vi "rmad aux data to file.vi"(1 "Avalanch JBV":T1(array[cluster]) {"A2 mean" format="%.1f"; "A1 mean" format="%.1f"; "A1 std" format="%.1f"; "A2 std" format="%.1f"}, 2 "aux_datadir":string, 3 "event_datadir":string, 5 "Avalanch Packets":T3(array[cluster]) {"A1 std" format="%.1g"; "A2 std" format="%.1g"; "A3 std" format="%.1g"; "A4 std" format="%.1g"}, 7 "vdv_datadir":string, 9 "last packet type":u8[](array[numeric]), 11 "error in":errorcluster, 12 "AUX data":T2(array[cluster]) {"batteri (V)" format="%.3g"; "temperatur (c)" format="%.1g"}, 13 "mac adresses":T4) -> (15 "error out":errorcluster)   [LabVIEW 2017]
panel:
  out "previous line in dat file":string
  out "last vdv record number":i32
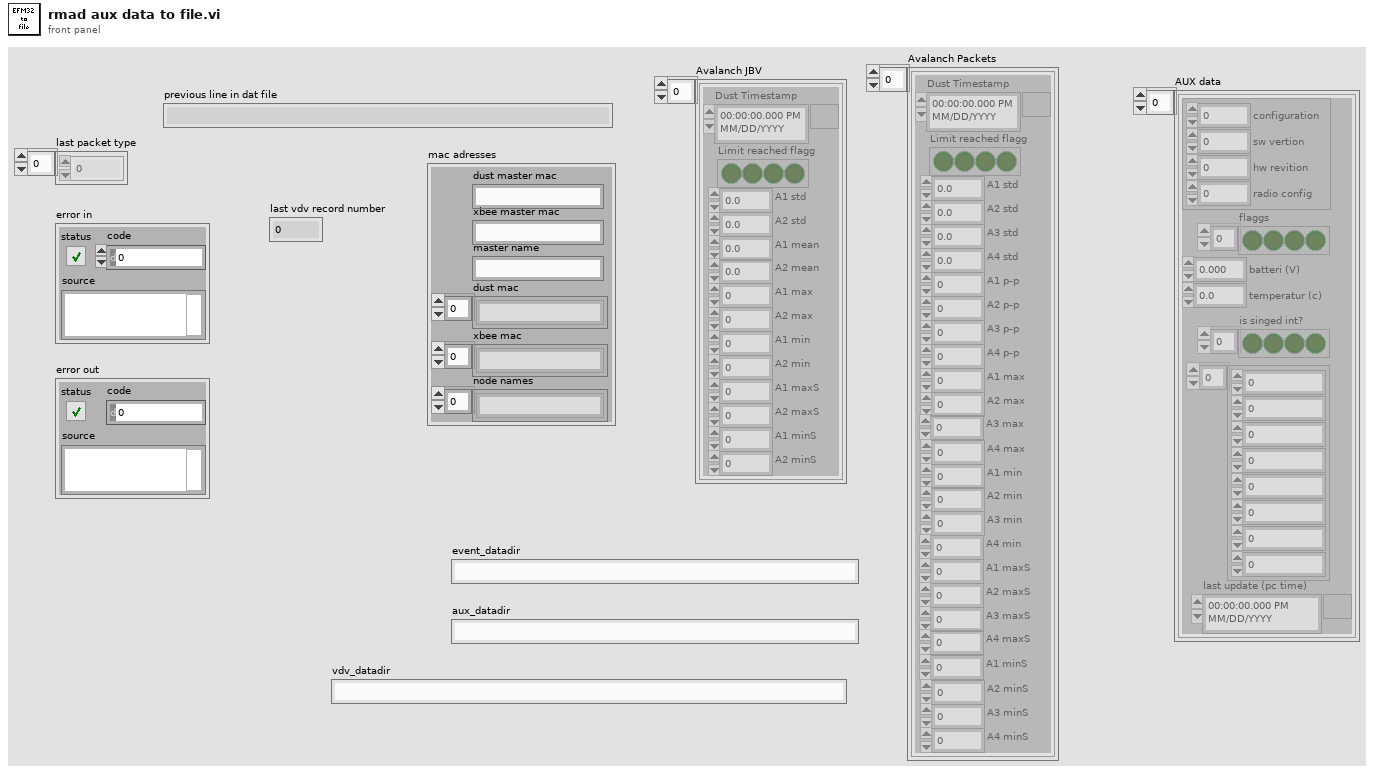
[diagram p1: front panel]
types:
  T1 = cluster{"Dust Timestamp":timestamp, "Limit reached flagg":bool[], "A1 std":sgl, "A2 std":sgl, "A1 mean":sgl, "A2 mean":sgl, "A1 max":i32, "A2 max":i32, "A1 min":i32, "A2 min":i32, "A1 maxS":u16, "A2 maxS":u16, "A1 minS":u16, "A2 minS":u16}[]
  T2 = cluster{cluster{"configuration":u8, "sw vertion":u8, "hw revition":u8, "radio config":u8}, "flaggs":bool[], "batteri (V)":dbl, "temperatur (c)":dbl, "is singed int?":bool[], dbl[], "last update (pc time)":timestamp}[]
  T3 = cluster{"Dust Timestamp":timestamp, "Limit reached flagg":bool[], "A1 std":sgl, "A2 std":sgl, "A3 std":sgl, "A4 std":sgl, "A1 p-p":sgl, "A2 p-p":sgl, "A3 p-p":sgl, "A4 p-p":sgl, "A1 max":u16, "A2 max":u16, "A3 max":u16, "A4 max":u16, "A1 min":u16, "A2 min":u16, "A3 min":u16, "A4 min":u16, "A1 maxS":u16, "A2 maxS":u16, "A3 maxS":u16, "A4 maxS":u16, "A1 minS":u16, "A2 minS":u16, "A3 minS":u16, "A4 minS":u16}[]
  T4 = cluster{"dust master mac":string, "xbee master mac":string, "master name":string, "dust mac":string[], "xbee mac":string[], "node names":string[]}
  T5 = enum16{"open", "replace", "create", "open or create", "replace or create", "replace or create with confirmation"}
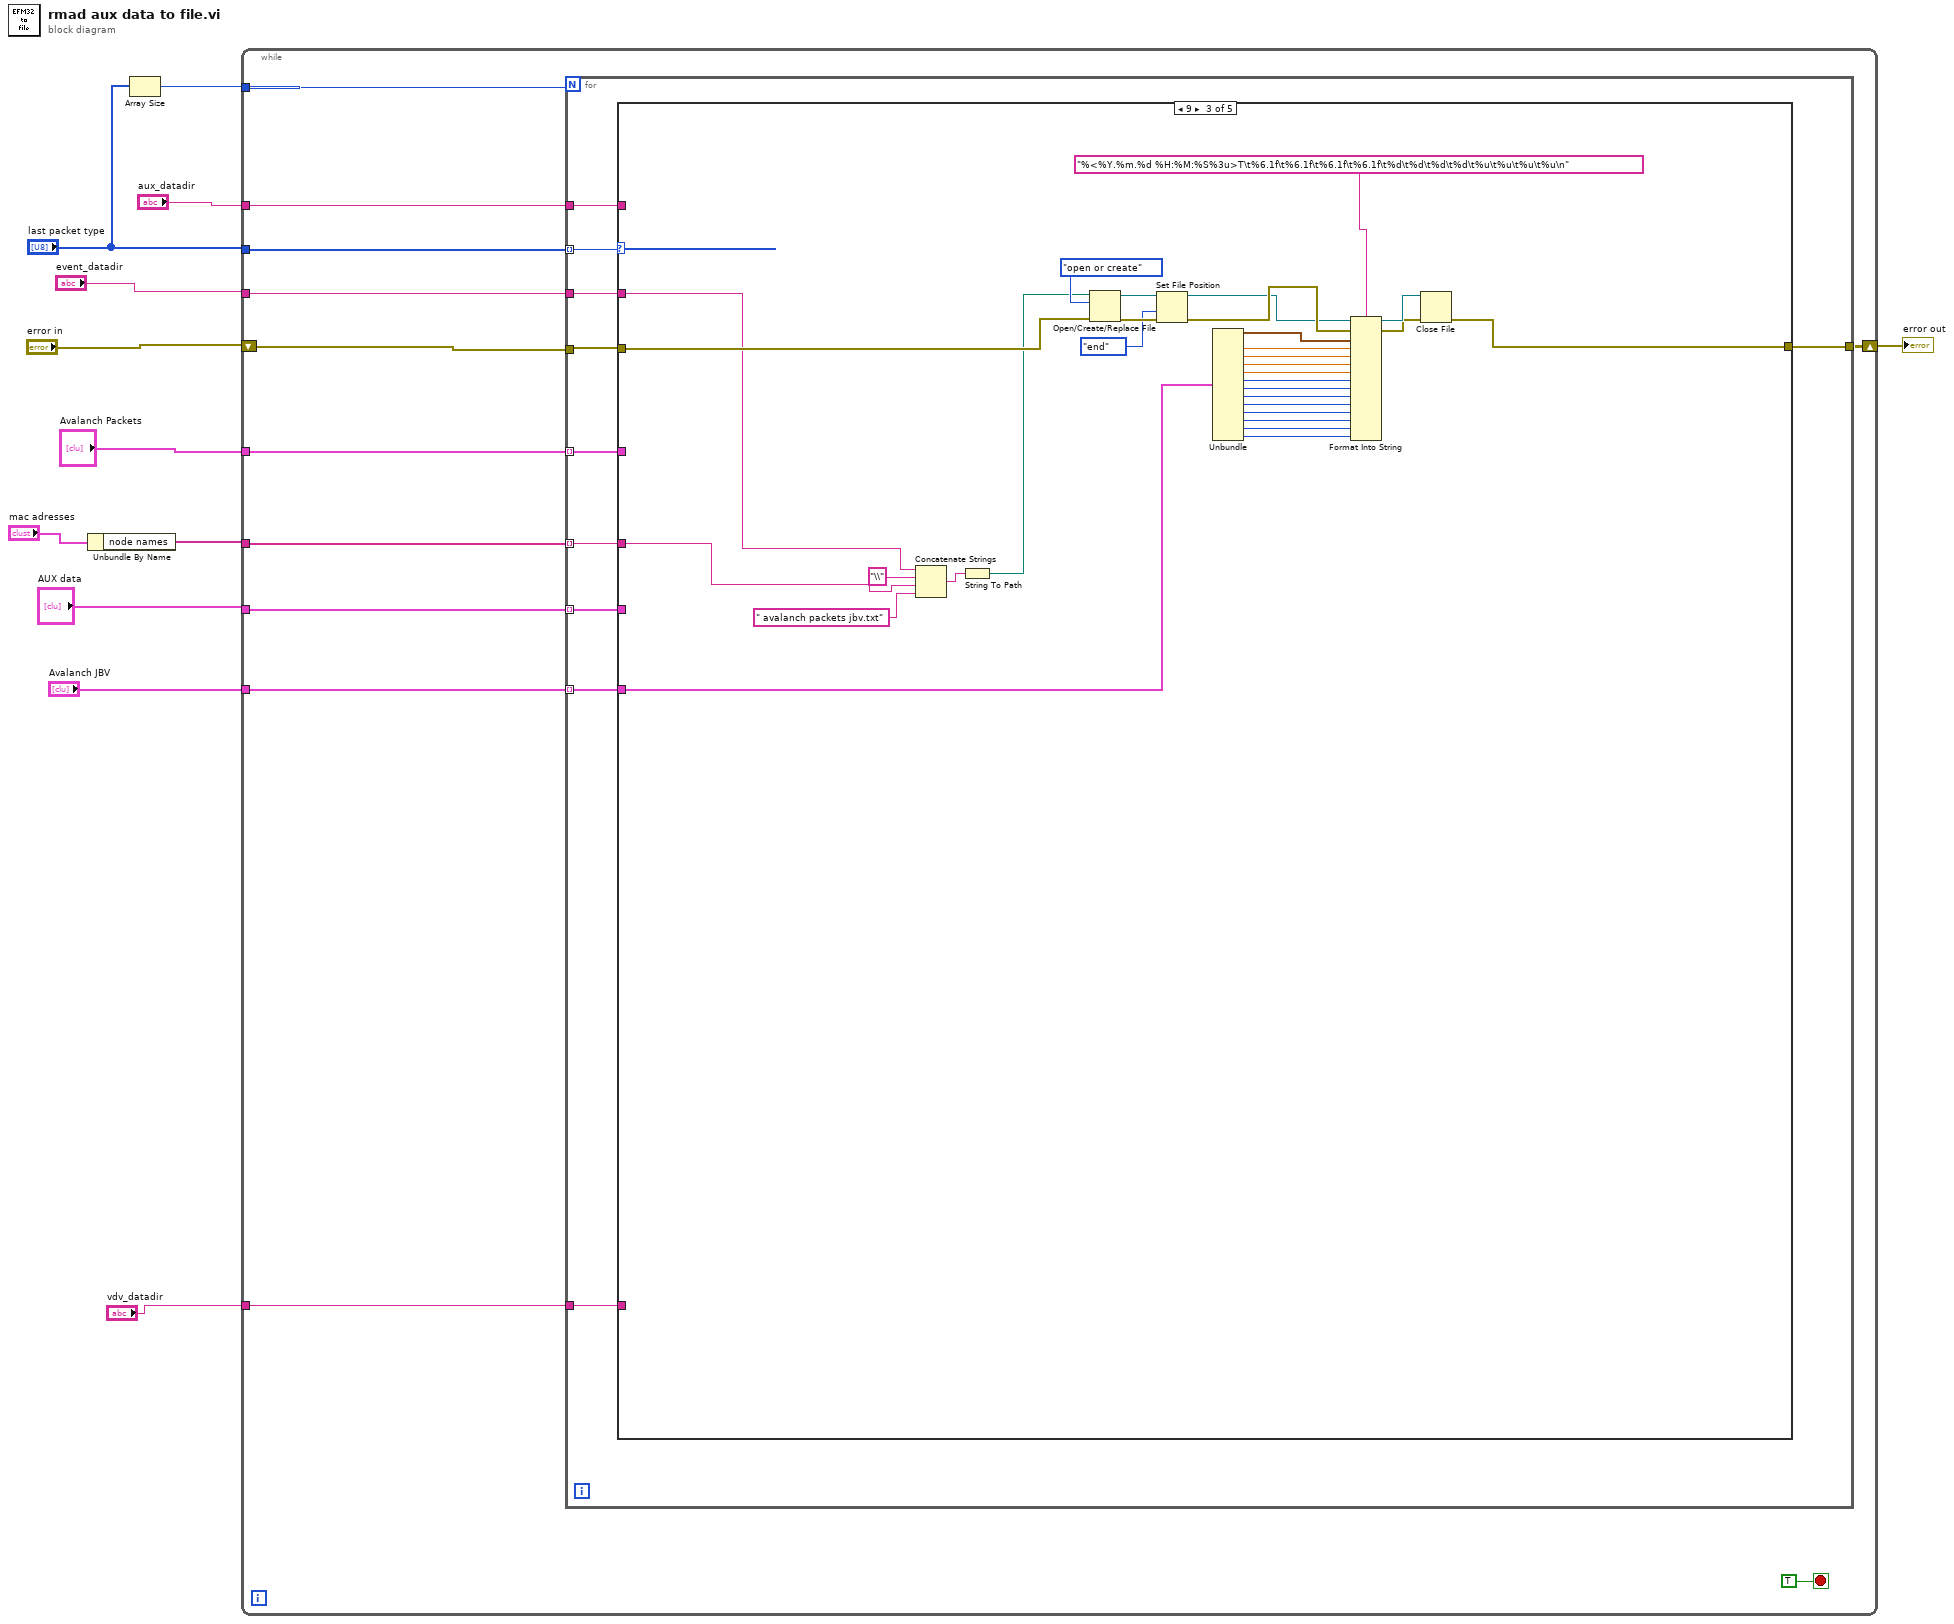
[diagram p0: block diagram]
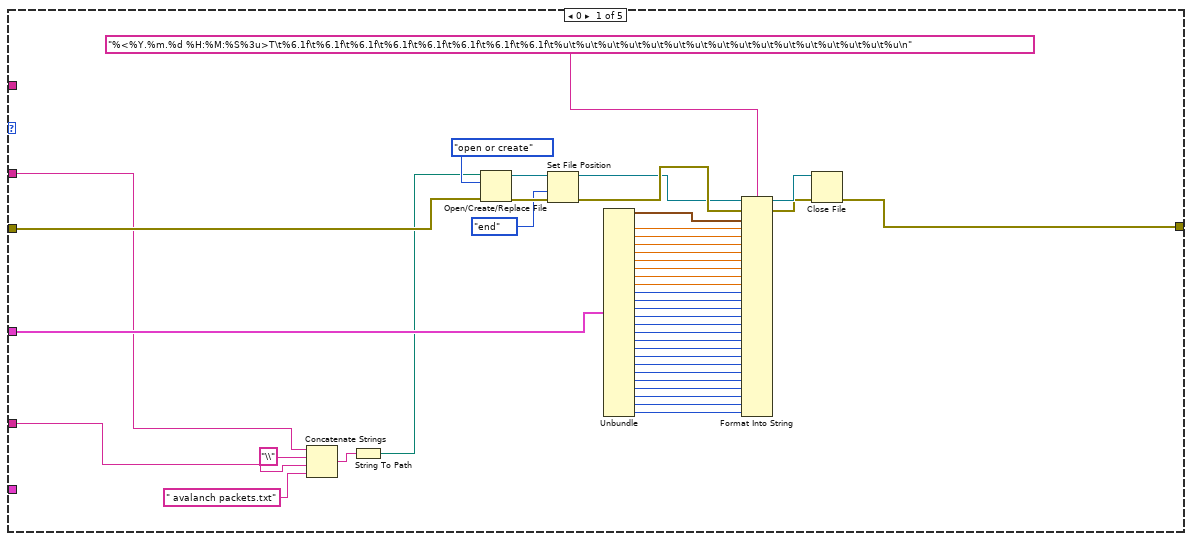
[diagram p2: hidden frame]
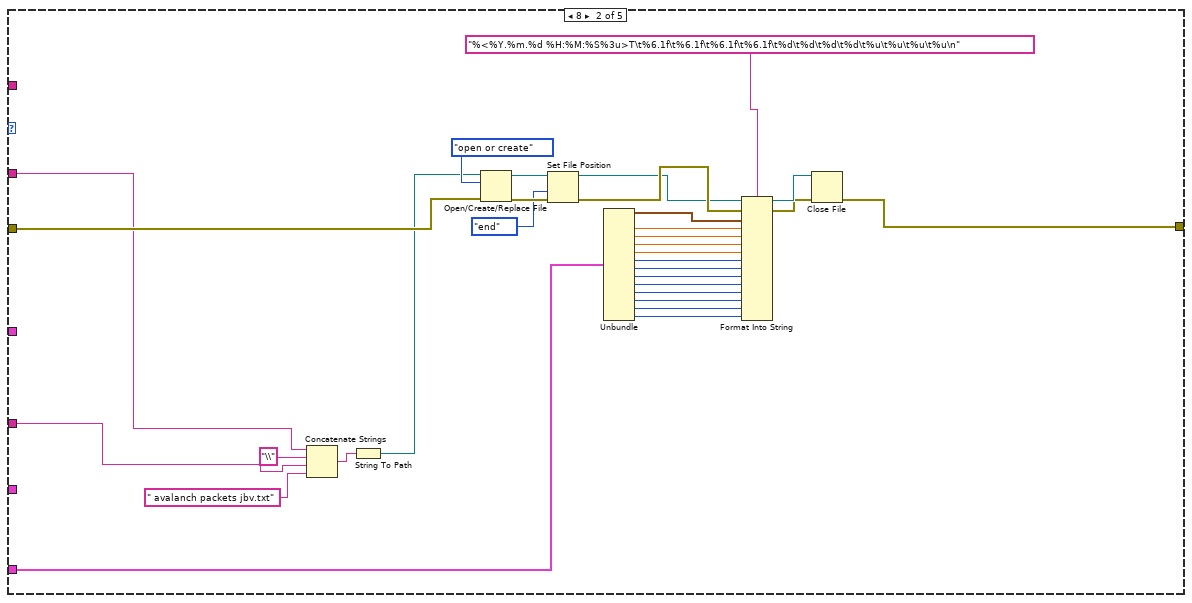
[diagram p3: hidden frame]
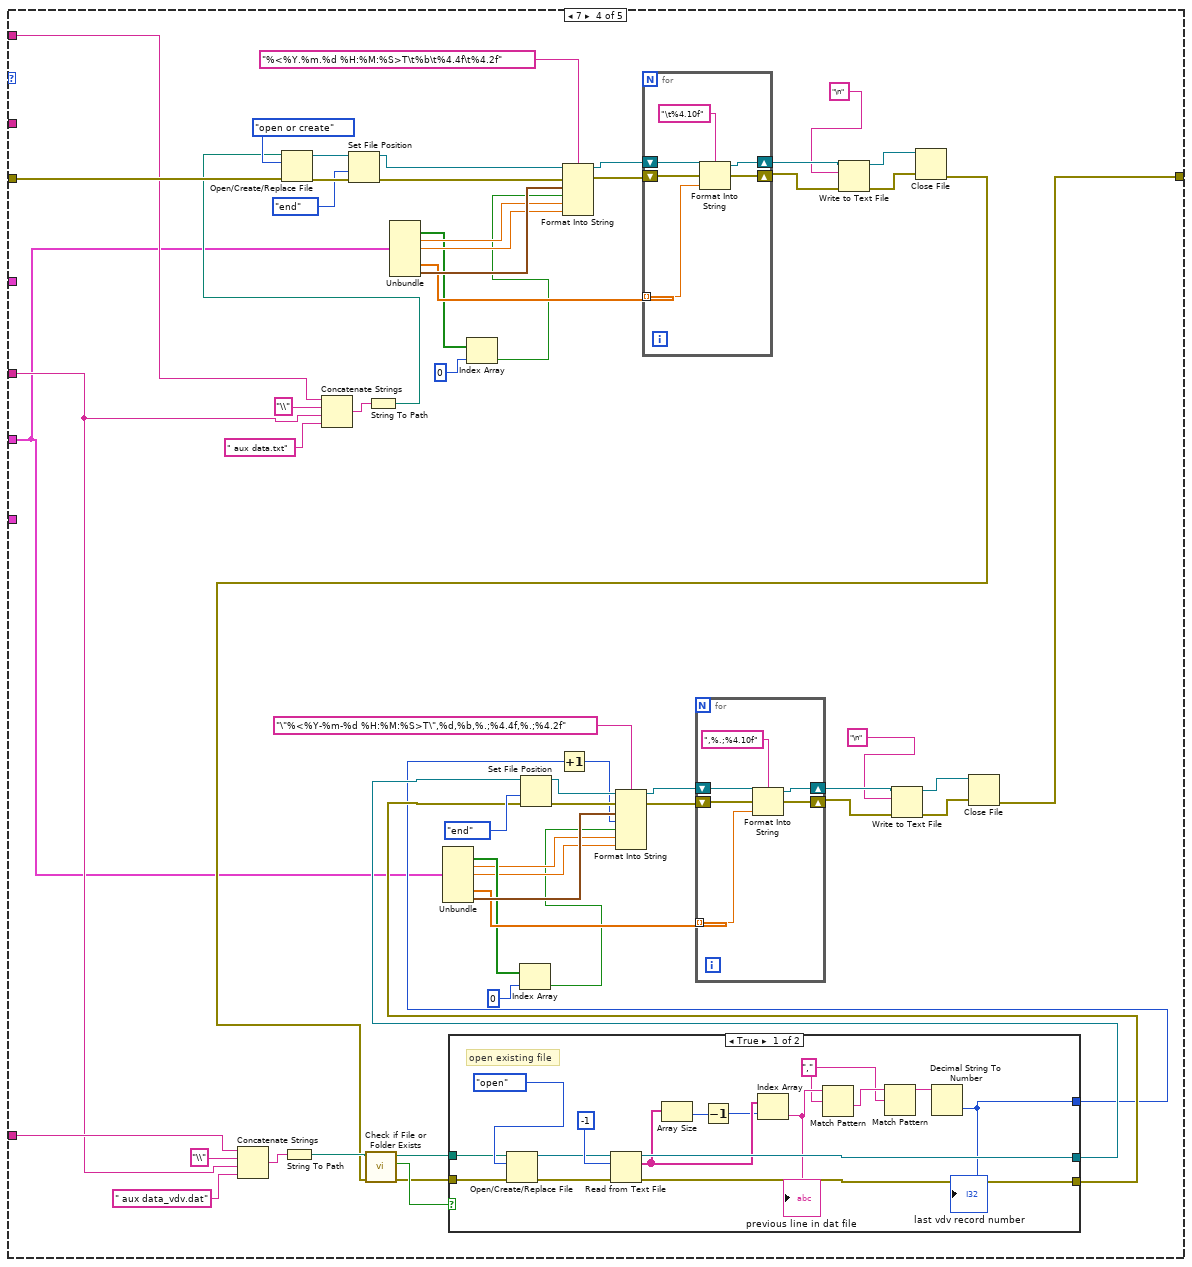
[diagram p4: hidden frame]
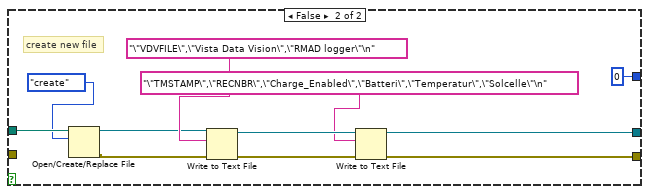
[diagram p5: hidden frame]
diagram:
  n1 = Unbundle By Name("mac adresses") -> ("node names"=w6:string[])
  n2 = Array Size(array="last packet type") -> (size(s)=w9:i32)
  n3 = while {
    tunnel: "event_datadir" -> [w22]
    tunnel: w9 -> [w15]
    tunnel: "last packet type" -> [w21]
    tunnel: w6 -> [w20]
    tunnel: "Avalanch Packets" -> [w19]
    tunnel: "AUX data" -> [w18]
    tunnel: "aux_datadir" -> [w17]
    shift-right: [w23] -> w11
    shift-left: "error in" -> [w24]
    tunnel: "Avalanch JBV" -> [w14]
    tunnel: "vdv_datadir" -> [w13]
    stop <- TRUE stop-if-true
    n4 = for {
      N: w15 -> [_]
      tunnel: w21 -> [w34] mode=indexing
      tunnel: w19 -> [w31] mode=indexing
      tunnel: w24 -> [w33]
      tunnel: [w27] -> w23
      tunnel: w22 -> [w32]
      tunnel: w20 -> [w29] mode=indexing
      tunnel: w18 -> [w30] mode=indexing
      tunnel: w17 -> [w28]
      tunnel: w14 -> [w26] mode=indexing
      tunnel: w13 -> [w25]
      n5 = case shown="9" w34 {
        tunnel: w31 -> [w77 _ _ _ _]
        tunnel: w33 -> [w72 w104 w135 w199 w240]
        tunnel: [w71 w103 w134 w143 w240] -> w27
        tunnel: w32 -> [w61 w93 w124 _ _]
        tunnel: w29 -> [w60 w92 w123 w141 _]
        tunnel: w30 -> [_ _ _ w140 _]
        tunnel: w28 -> [_ _ _ w174 _]
        tunnel: w26 -> [_ w78 w109 _ _]
        tunnel: w25 -> [_ _ _ w142 _]
        frame 0 {
          n6 = Concatenate Strings(w61, "\\" ("string"), w60, " avalanch packets.txt" ("string")) -> (w63:string)
          n7 = String To Path(string=w63) -> (path=w59:path)
          n8 = Open/Create/Replace File(file path (use dialog)=w59, error in=w72, operation (0:open)=T5."open or create") -> (refnum out=w74:refnum<file>, error out=w75:errorcluster)  [unwired: 3 in, 1 out]
          n9 = Set File Position(refnum=w74, from (0:start)=enum16{"start", "end", "current"}."end", error in=w75) -> (refnum out=w69:refnum<file>, error out=w70:errorcluster)  [unwired: 1 in]
          n10 = Unbundle(w77) -> ("Dust Timestamp"=w65:timestamp, "A1 std"=w58:sgl, "A2 std"=w57:sgl, "A3 std"=w56:sgl, "A4 std"=w55:sgl, "A1 p-p"=w54:sgl, "A2 p-p"=w53:sgl, "A3 p-p"=w52:sgl, "A4 p-p"=w51:sgl, "A1 max"=w50:u16, "A2 max"=w49:u16, "A3 max"=w48:u16, "A4 max"=w47:u16, "A1 min"=w46:u16, "A2 min"=w45:u16, "A3 min"=w44:u16, "A4 min"=w43:u16, "A1 maxS"=w42:u16, "A2 maxS"=w41:u16, "A3 maxS"=w40:u16, "A4 maxS"=w39:u16, "A1 minS"=w38:u16, "A2 minS"=w37:u16, "A3 minS"=w36:u16, "A4 minS"=w35:u16)  [unwired: 1 out]
          n11 = Format Into String(format string="%<%Y.%m.%d %H:%M:%S%3u>T\t%6.1f\t%6.1f\t%6.1f\t%6.1f\t%6.1f\t%6.1f\t%6.1f\t%6.1f\t%u\t%u\t%u\t%u\t%u\t%u\t%u\t%u\t%u\t%u\t%u\t%u\t%u\t%u\t%u\t%u\n", initial string=w69, error in=w70, w65, w58, w57, w56, w55, w54, w53, w52, w51, w50, w49, w48, w47, w46, w45, w44, w43, w42, w41, w40, w39, w38, w37, w36, w35) -> (resulting string=w67:refnum<file>, error out=w66:errorcluster)
          n12 = Close File(refnum=w67, error in=w66) -> (error out=w71:errorcluster)  [unwired: 1 out]
        }
        frame 8 {
          n13 = Concatenate Strings(w93, "\\" ("string"), w92, " avalanch packets jbv.txt" ("string")) -> (w95:string)
          n14 = String To Path(string=w95) -> (path=w91:path)
          n15 = Open/Create/Replace File(file path (use dialog)=w91, error in=w104, operation (0:open)=T5."open or create") -> (refnum out=w106:refnum<file>, error out=w107:errorcluster)  [unwired: 3 in, 1 out]
          n16 = Set File Position(refnum=w106, from (0:start)=enum16{"start", "end", "current"}."end", error in=w107) -> (refnum out=w101:refnum<file>, error out=w102:errorcluster)  [unwired: 1 in]
          n17 = Unbundle(w78) -> ("Dust Timestamp"=w97:timestamp, "A1 std"=w90:sgl, "A2 std"=w89:sgl, "A1 mean"=w88:sgl, "A2 mean"=w87:sgl, "A1 max"=w86:i32, "A2 max"=w85:i32, "A1 min"=w84:i32, "A2 min"=w83:i32, "A1 maxS"=w82:u16, "A2 maxS"=w81:u16, "A1 minS"=w80:u16, "A2 minS"=w79:u16)  [unwired: 1 out]
          n18 = Format Into String(format string="%<%Y.%m.%d %H:%M:%S%3u>T\t%6.1f\t%6.1f\t%6.1f\t%6.1f\t%d\t%d\t%d\t%d\t%u\t%u\t%u\t%u\n", initial string=w101, error in=w102, w97, w90, w89, w88, w87, w86, w85, w84, w83, w82, w81, w80, w79) -> (resulting string=w99:refnum<file>, error out=w98:errorcluster)
          n19 = Close File(refnum=w99, error in=w98) -> (error out=w103:errorcluster)  [unwired: 1 out]
        }
        frame 9 {
          n20 = Concatenate Strings(w124, "\\" ("string"), w123, " avalanch packets jbv.txt" ("string")) -> (w126:string)
          n21 = String To Path(string=w126) -> (path=w122:path)
          n22 = Open/Create/Replace File(file path (use dialog)=w122, error in=w135, operation (0:open)=T5."open or create") -> (refnum out=w137:refnum<file>, error out=w138:errorcluster)  [unwired: 3 in, 1 out]
          n23 = Set File Position(refnum=w137, from (0:start)=enum16{"start", "end", "current"}."end", error in=w138) -> (refnum out=w132:refnum<file>, error out=w133:errorcluster)  [unwired: 1 in]
          n24 = Unbundle(w109) -> ("Dust Timestamp"=w128:timestamp, "A1 std"=w121:sgl, "A2 std"=w120:sgl, "A1 mean"=w119:sgl, "A2 mean"=w118:sgl, "A1 max"=w117:i32, "A2 max"=w116:i32, "A1 min"=w115:i32, "A2 min"=w114:i32, "A1 maxS"=w113:u16, "A2 maxS"=w112:u16, "A1 minS"=w111:u16, "A2 minS"=w110:u16)  [unwired: 1 out]
          n25 = Format Into String(format string="%<%Y.%m.%d %H:%M:%S%3u>T\t%6.1f\t%6.1f\t%6.1f\t%6.1f\t%d\t%d\t%d\t%d\t%u\t%u\t%u\t%u\n", initial string=w132, error in=w133, w128, w121, w120, w119, w118, w117, w116, w115, w114, w113, w112, w111, w110) -> (resulting string=w130:refnum<file>, error out=w129:errorcluster)
          n26 = Close File(refnum=w130, error in=w129) -> (error out=w134:errorcluster)  [unwired: 1 out]
        }
        frame 7 {
          n27 = Concatenate Strings(w142, "\\" ("string"), w141, " aux data_vdv.dat" ("string")) -> (w168:string)
          n28 = String To Path(string=w168) -> (path=w151:path)
          n29 = Concatenate Strings(w174, "\\" ("string"), w141, " aux data.txt" ("string")) -> (w191:string)
          n30 = String To Path(string=w191) -> (path=w189:path)
          n31 = Open/Create/Replace File(file path (use dialog)=w189, error in=w199, operation (0:open)=T5."open or create") -> (refnum out=w195:refnum<file>, error out=w197:errorcluster)  [unwired: 3 in, 1 out]
          n32 = Set File Position(refnum=w195, from (0:start)=enum16{"start", "end", "current"}."end", error in=w197) -> (refnum out=w194:refnum<file>, error out=w196:errorcluster)  [unwired: 1 in]
          n33 = Unbundle(w140) -> ("flaggs"=w177:bool[], "batteri (V)"=w187:dbl, "temperatur (c)"=w186:dbl, w185:dbl[], "last update (pc time)"=w188:timestamp)  [unwired: 2 out]
          n34 = Unbundle(w140) -> ("flaggs"=w157:bool[], "batteri (V)"=w148:dbl, "temperatur (c)"=w149:dbl, w165:dbl[], "last update (pc time)"=w166:timestamp)  [unwired: 2 out]
          n35 = Index Array(array=w177, index=0) -> (element=w175:bool)
          n36 = Index Array(array=w157, index=0) -> (element=w147:bool)
          n37 = Format Into String(format string="%<%Y.%m.%d %H:%M:%S>T\t%b\t%4.4f\t%4.2f", initial string=w194, error in=w196, w188, w175, w187, w186) -> (resulting string=w183:refnum<file>, error out=w184:errorcluster)
          n38 = for {
            tunnel: w185 -> [w235] mode=indexing
            shift-right: [w236] -> w182
            shift-left: w183 -> [w237]
            shift-right: [w238] -> w180
            shift-left: w184 -> [w239]
            n39 = Format Into String(format string="\t%4.10f", initial string=w237, error in=w239, w235) -> (resulting string=w236:refnum<file>, error out=w238:errorcluster)
          }
          n40 = Write to Text File(file (use dialog)=w182, text="\n" ("format string"), error in=w180) -> (refnum out=w181:refnum<file>, error out=w179:errorcluster)  [unwired: 1 in, 1 out]
          n41 = Close File(refnum=w181, error in=w179) -> (error out=w144:errorcluster)  [unwired: 1 out]
          n42 = call <vilib>:"Check if File or Folder Exists.vi"("error in (no error)"=w144, "path"=w151) -> ("error out"=w154:errorcluster, "file or folder exists?"=w155:bool, "dup path"=w150:path)  [unwired: 7 in]
          n43 = case shown="True" w155 {
            tunnel: w150 -> [w214 w227]
            tunnel: [w213 w219] -> w153
            tunnel: [w212 w218] -> w152
            tunnel: w154 -> [w216 _]
            tunnel: [w201 0] -> w146
            frame True {
              w203 = "," ("regular expression")
              # "open existing file"
              n44 = Open/Create/Replace File(file path (use dialog)=w214, error in=w216, operation (0:open)=T5."open") -> (refnum out=w209:refnum<file>, error out=w210:errorcluster)  [unwired: 3 in, 1 out]
              n45 = Read from Text File(file (use dialog)=w209, count=-1, error in=w210) -> (refnum out=w212:refnum<file>, text=w208:string[], error out=w213:errorcluster)  [unwired: 1 in, 1 out]
              n46 = Array Size(array=w208) -> (size(s)=w207:i32)
              n47 = Decrement(x=w207) -> (x-1=w206:i32)
              n48 = Index Array(array=w208, index=w206) -> (element=w205:string)
              "previous line in dat file" <- w205
              n49 = Match Pattern(string=w205, regular expression=w203) -> (after substring=w204:string)  [unwired: 1 in, 3 out]
              n50 = Match Pattern(string=w204, regular expression=w203) -> (before substring=w202:string)  [unwired: 1 in, 3 out]
              n51 = Decimal String To Number(string=w202) -> (number=w201:i32)  [unwired: 2 in, 1 out]
              "last vdv record number" <- w201
            }
            frame False {
              # "create new file"
              n52 = Open/Create/Replace File(file path (use dialog)=w227, operation (0:open)=T5."create") -> (refnum out=w223:refnum<file>, error out=w224:errorcluster)  [unwired: 4 in, 1 out]
              n53 = Write to Text File(file (use dialog)=w223, text="\"VDVFILE\",\"Vista Data Vision\",\"RMAD logger\"\n" ("format string"), error in=w224) -> (refnum out=w221:refnum<file>, error out=w222:errorcluster)  [unwired: 1 in, 1 out]
              n54 = Write to Text File(file (use dialog)=w221, text="\"TMSTAMP\",\"RECNBR\",\"Charge_Enabled\",\"Batteri\",\"Temperatur\",\"Solcelle\"\n" ("format string"), error in=w222) -> (refnum out=w218:refnum<file>, error out=w219:errorcluster)  [unwired: 1 in, 1 out]
            }
          }
          n55 = Set File Position(refnum=w152, from (0:start)=enum16{"start", "end", "current"}."end", error in=w153) -> (refnum out=w171:refnum<file>, error out=w172:errorcluster)  [unwired: 1 in]
          n56 = Increment(x=w146) -> (x+1=w145:i32)
          n57 = Format Into String(format string="\"%<%Y-%m-%d %H:%M:%S>T\",%d,%b,%.;%4.4f,%.;%4.2f", initial string=w171, error in=w172, w166, w145, w147, w148, w149) -> (resulting string=w163:refnum<file>, error out=w164:errorcluster)
          n58 = for {
            tunnel: w165 -> [w229] mode=indexing
            shift-right: [w230] -> w162
            shift-left: w163 -> [w231]
            shift-right: [w232] -> w160
            shift-left: w164 -> [w233]
            n59 = Format Into String(format string=",%.;%4.10f", initial string=w231, error in=w233, w229) -> (resulting string=w230:refnum<file>, error out=w232:errorcluster)
          }
          n60 = Write to Text File(file (use dialog)=w162, text="\n" ("format string"), error in=w160) -> (refnum out=w161:refnum<file>, error out=w159:errorcluster)  [unwired: 1 in, 1 out]
          n61 = Close File(refnum=w161, error in=w159) -> (error out=w143:errorcluster)  [unwired: 1 out]
        }
        frame 100, Default {
        }
      }
    }
  }
  "error out" <- w11
